vi "Traffic lights.vi"() -> ()   [LabVIEW 2018]
panel:
  out "GREEN":bool
  out "YELLOW":bool
  out "RED":bool
  out "GREEN":bool
  out "YELLOW":bool
  out "RED":bool
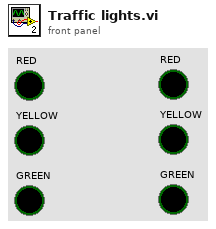
[diagram p1: front panel]
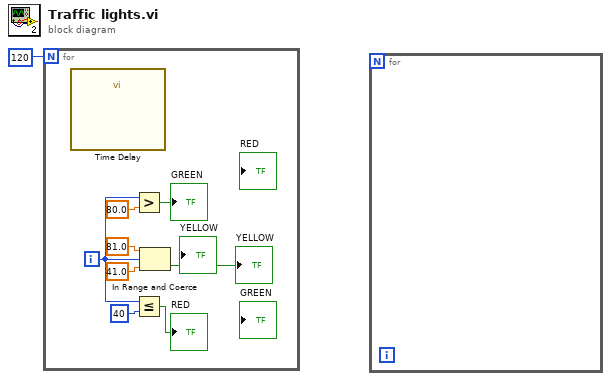
[diagram p0: block diagram]
diagram:
  n1 = for {
    N: 120 -> [_]
    i -> [w2]
    n2 = call "Time Delay"() -> ()  [unwired: 11 in, 1 out]
    n3 = Greater?(x=w2, y=80.0) -> (0:→"GREEN":bool)
    n4 = Less Or Equal?(x=w2, y=40) -> (x <= y?=→"RED":bool)
    n5 = In Range and Coerce(upper limit=81.0, x=w2, lower limit=41.0) -> (In Range?=→"YELLOW":bool)  [unwired: 1 out]
  }
  n6 = for {
  }
